vi "Unpack U32 Value.vi"(11 "U32ValueMsg in":refnum<class "U32ValueMsg.lvclass">) -> (2 "Value":u32, 3 "Name":string)   [LabVIEW 2015, in "ActorAutoRegistration.lvlib" / "U32ValueMsg.lvclass"]
uses:
  U32ValueMsg.lvclass
  U32ValueMsg.lvclass/U32ValueMsg.ctl
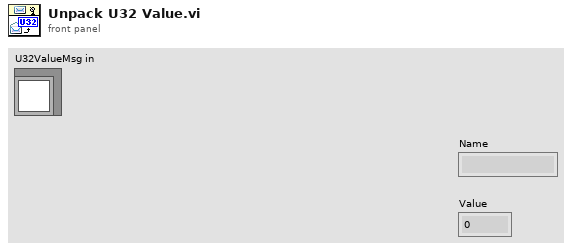
[diagram p1: front panel]
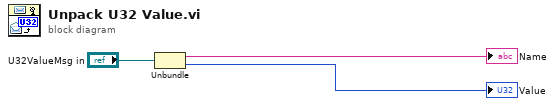
[diagram p0: block diagram]
diagram:
  n1 = Unbundle("U32ValueMsg in") -> (→"Name":string, →"Value":u32)
